vi "List Users.vi"(7 "PwdMgr in":refnum<class "PwdMgr.lvclass">, 8 "error in (no error)":errorcluster) -> (0 "error out":errorcluster, 3 "Array":T1[](array[typedef]))   [LabVIEW 2020, in "Login-UI.lvlib" / "PwdMgr.lvclass"]
uses:
  PwdMgr.lvclass
  _Typedef/User-Info.ctl
  _Typedef/User-Role.ctl
  Login-UI.lvlib
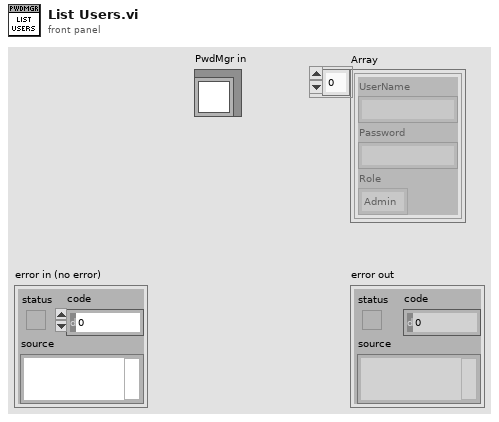
[diagram p1: front panel]
types:
  T1 = typedef "Login-UI.lvlib/User-Info.ctl" = cluster{"UserName":string, "Password":string, "Role":T2}
  T2 = typedef "Login-UI.lvlib/User-Role.ctl" = enum16{"INVALID", "Operator", "Engineer", "Admin", "Anonymous"}
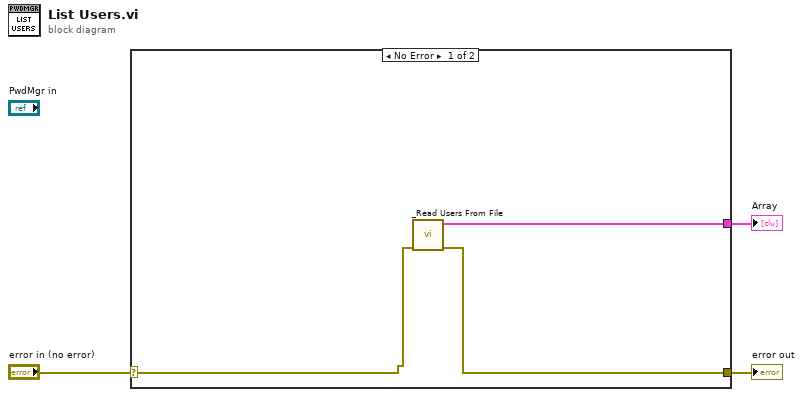
[diagram p0: block diagram]
diagram:
  n1 = case shown="No Error" "error in (no error)" {
    selector: "error in (no error)" -> [w6 w7]
    tunnel: [w5 w7] -> w2
    tunnel: [w4 _] -> w1
    frame No Error {
      n2 = call "_Read Users From File.vi"("Error in"=w6) -> ("Error out"=w5:errorcluster, "Array"=w4:T1[])  [unwired: 9 in]
    }
    frame Error {
    }
  }
  "error out" <- w2
  "Array" <- w1
